vi "Set Defaults.vi"(11 "NewEntityTemplate in":refnum<class "NewEntityTemplate.lvclass">) -> (3 "NewEntityTemplate out":refnum<class "NewEntityTemplate.lvclass">)   [LabVIEW 2020, in "Conditum-Tools.lvlib" / "NewEntityTemplate.lvclass"]
uses:
  NewEntityTemplate.lvclass
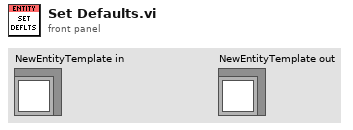
[diagram p1: front panel]
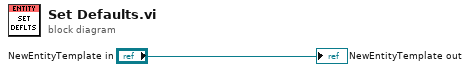
[diagram p0: block diagram]
diagram:
  "NewEntityTemplate out" <- "NewEntityTemplate in"
